vi "Set Wheel Parameter by Name.vi"(8 "error in (no error)":errorcluster, 9 "parameter value":variant, 10 "parameter name":string, 11 "wheel in":refnum<class "NI_Robotics_Caster Wheel.lvclass">) -> (0 "error out":errorcluster, 1 "set?":bool, 3 "wheel out":refnum<class "NI_Robotics_Caster Wheel.lvclass">)   [LabVIEW 2017, in "NI_Robotics_Caster Wheel.lvclass"]
uses:
  <vilib>/robotics/Steering/Caster Wheel/NI_Robotics_Caster Wheel.lvclass
  <vilib>/robotics/Steering/Caster Wheel/NI_Robotics_Caster Wheel.lvclass/NI_Robotics_Caster Wheel.ctl
  <vilib>/robotics/Actuation/Motor Communication/NI_Robotics_Motor Communication.lvclass
  <vilib>/robotics/Steering/Wheel/NI_Robotics_Wheel.lvclass
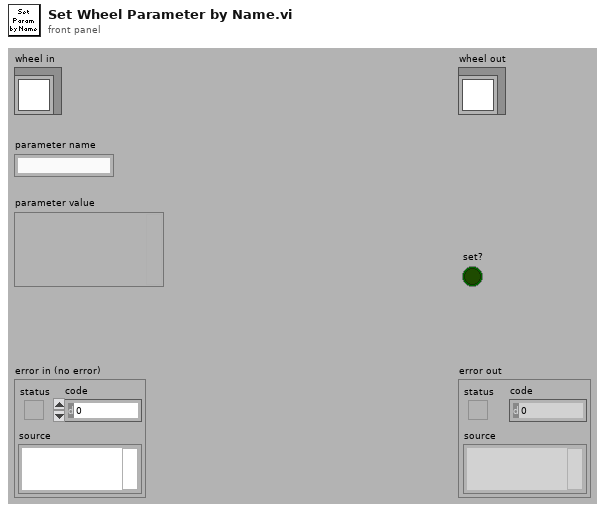
[diagram p1: front panel]
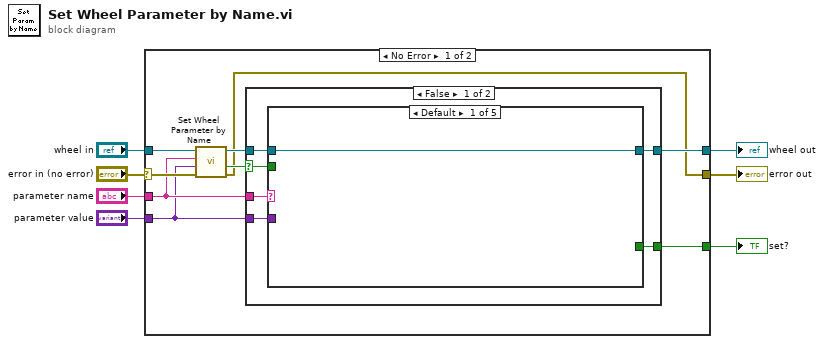
[diagram p0: block diagram]
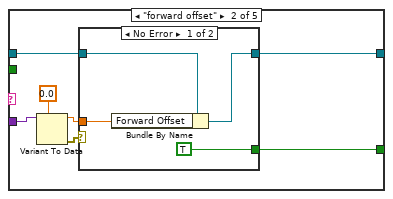
[diagram p2: hidden frame]
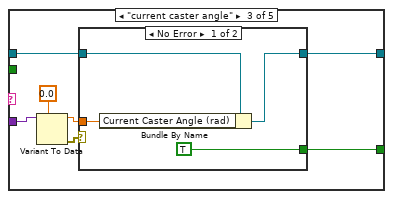
[diagram p4: hidden frame]
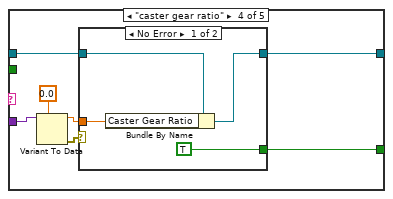
[diagram p6: hidden frame]
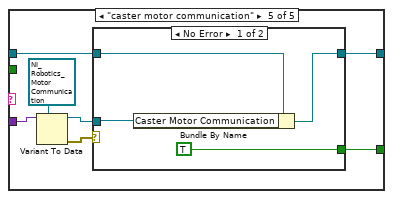
[diagram p8: hidden frame]
diagram:
  n1 = case shown="No Error" "error in (no error)" {
    selector: "error in (no error)" -> [w15 w74]
    tunnel: "parameter value" -> [w11 _]
    tunnel: "parameter name" -> [w12 _]
    tunnel: "wheel in" -> [w16 w75]
    tunnel: [w10 w75] -> w3
    tunnel: [w9 _] -> w2
    tunnel: [w8 w74] -> w1
    frame No Error {
      n2 = call-parent "Set Wheel Parameter by Name.vi"("error in (no error)"=w15, "parameter value"=w11, "parameter name"=w12, "wheel in"=w16) -> ("error out"=w8:errorcluster, "set?"=w13:bool, "wheel out"=w14:refnum<class "NI_Robotics_Caster Wheel.lvclass">)  [unwired: 5 in]
      n3 = case shown="False" w13 {
        selector: w13 -> [w19 w72]
        tunnel: w14 -> [w22 w73]
        tunnel: [w20 w73] -> w10
        tunnel: w12 -> [w21 _]
        tunnel: [w18 w72] -> w9
        tunnel: w11 -> [w17 _]
        frame False {
          n4 = case shown="Default" w21 {
            tunnel: w22 -> [w23 w30 w42 w54 w66]
            tunnel: [w23 w29 w41 w53 w65] -> w20
            tunnel: w19 -> [_ _ _ _ _]
            tunnel: [_ w24 w36 w48 w61] -> w18
            tunnel: w17 -> [_ w28 w40 w52 w64]
            frame Default {
            }
            frame "forward offset" {
              n5 = Variant To Data(type=0.0 ("Steering Gear Ratio"), Variant=w28) -> (data=w25:dbl, error out=w26:errorcluster)  [unwired: 1 in]
              n6 = case shown="No Error" w26 {
                tunnel: w30 -> [w34 w35]
                tunnel: [w33 w35] -> w29
                tunnel: w25 -> [w32 _]
                tunnel: [TRUE _] -> w24
                frame No Error {
                  n7 = Bundle By Name(cluster=w34, "Forward Offset"=w32) -> (w33:refnum<class "NI_Robotics_Caster Wheel.lvclass">)
                }
                frame Error {
                }
              }
            }
            frame "current caster angle" {
              n8 = Variant To Data(type=0.0 ("Steering Gear Ratio"), Variant=w40) -> (data=w37:dbl, error out=w38:errorcluster)  [unwired: 1 in]
              n9 = case shown="No Error" w38 {
                tunnel: w42 -> [w46 w47]
                tunnel: [w45 w47] -> w41
                tunnel: w37 -> [w44 _]
                tunnel: [TRUE _] -> w36
                frame No Error {
                  n10 = Bundle By Name(cluster=w46, "Current Caster Angle (rad)"=w44) -> (w45:refnum<class "NI_Robotics_Caster Wheel.lvclass">)
                }
                frame Error {
                }
              }
            }
            frame "caster gear ratio" {
              n11 = Variant To Data(type=0.0 ("Steering Gear Ratio"), Variant=w52) -> (data=w49:dbl, error out=w50:errorcluster)  [unwired: 1 in]
              n12 = case shown="No Error" w50 {
                tunnel: w54 -> [w58 w59]
                tunnel: [w57 w59] -> w53
                tunnel: w49 -> [w56 _]
                tunnel: [TRUE _] -> w48
                frame No Error {
                  n13 = Bundle By Name(cluster=w58, "Caster Gear Ratio"=w56) -> (w57:refnum<class "NI_Robotics_Caster Wheel.lvclass">)
                }
                frame Error {
                }
              }
            }
            frame "caster motor communication" {
              n14 = Variant To Data(type=refnum<class "NI_Robotics_Motor Communication.lvclass"> refnum ("Steering Motor Communication"), Variant=w64) -> (data=w62:refnum<class "NI_Robotics_Motor Communication.lvclass">, error out=w63:errorcluster)  [unwired: 1 in]
              n15 = case shown="No Error" w63 {
                tunnel: w66 -> [w70 w71]
                tunnel: [w69 w71] -> w65
                tunnel: w62 -> [w67 _]
                tunnel: [TRUE _] -> w61
                frame No Error {
                  n16 = Bundle By Name(cluster=w70, "Caster Motor Communication"=w67) -> (w69:refnum<class "NI_Robotics_Caster Wheel.lvclass">)
                }
                frame Error {
                }
              }
            }
          }
        }
        frame True {
        }
      }
    }
    frame Error {
    }
  }
  "error out" <- w1
  "wheel out" <- w3
  "set?" <- w2
